vi "Write Meas Write registers.vi"(10 "Meas Write registers":T1(array[cluster]) {"Write Data Array" format="%.0x"}, 11 "Toggle 8 (niDig) in":refnum<class "Toggle 8 (niDig).lvclass">) -> (3 "Toggle 8 (niDig) out":refnum<class "Toggle 8 (niDig).lvclass">)   [LabVIEW 2020, in "Toggle 8 (niDig).lvclass"]
uses:
  Toggle 8 (niDig).lvclass
  Toggle 8 (niDig).lvclass/Toggle 8 (niDig).ctl
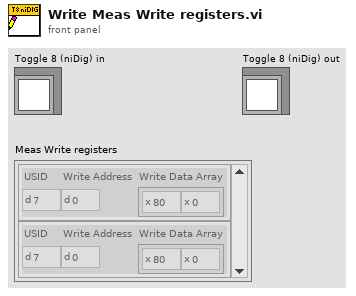
[diagram p1: front panel]
types:
  T1 = cluster{"USID":u8, "Write Address":u8, "Write Data Array":u8[]}[]
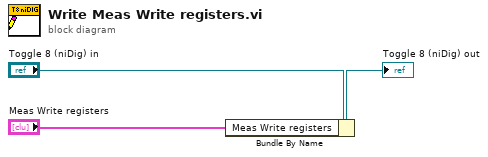
[diagram p0: block diagram]
diagram:
  n1 = Bundle By Name(cluster="Toggle 8 (niDig) in", "Meas Write registers"="Meas Write registers") -> (→"Toggle 8 (niDig) out":refnum<class "Toggle 8 (niDig).lvclass">)
